vi "sub_ofdm_simple_delayed_mult_CFO_sync_single.vi"(8 "CP length":i32=64, 9 "FFT size":i32=256, 11 "time samples":cdb[](array[numeric])) -> (3 "sync ofdm symbol":cdb[](array[numeric]))   [LabVIEW 2014]
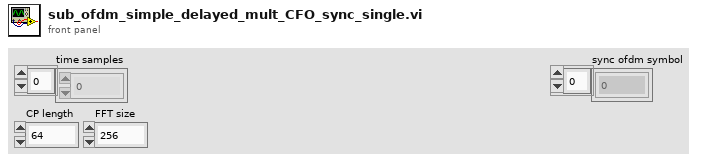
[diagram p1: front panel]
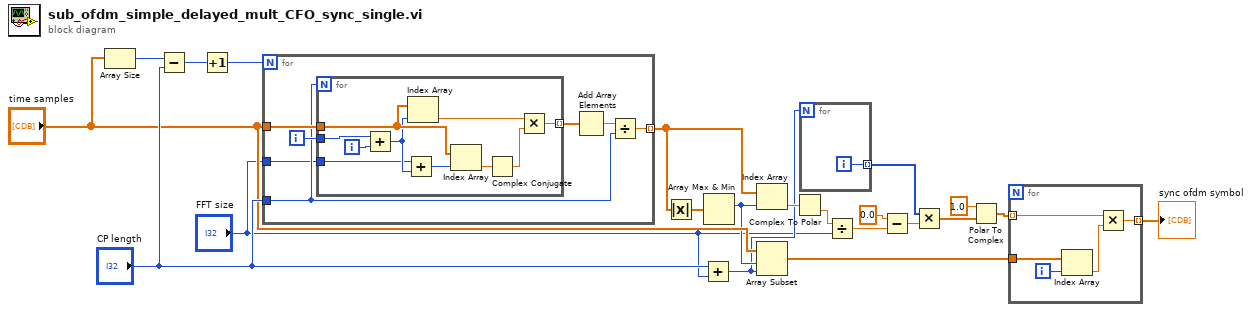
[diagram p0: block diagram]
diagram:
  n1 = Array Size(array="time samples") -> (size(s)=w17:i32)
  n2 = Subtract(x=w17, y="CP length") -> (x-y=w16:i32)
  n3 = Increment(x=w16) -> (x+1=w15:i32)
  n4 = for {
    N: w15 -> [_]
    tunnel: "CP length" -> [w26]
    tunnel: "time samples" -> [w28]
    tunnel: [w23] -> w20 mode=indexing
    tunnel: "FFT size" -> [w22]
    i -> [w27]
    n5 = for {
      N: w26 -> [_]
      tunnel: w28 -> [w34]
      tunnel: w27 -> [w38]
      tunnel: [w30] -> w24 mode=indexing
      tunnel: w22 -> [w29]
      i -> [w37]
      n6 = Add(x=w38, y=w37) -> (x+y=w33:i32)
      n7 = Add(x=w29, y=w33) -> (x+y=w36:i32)
      n8 = Index Array(array=w34, index=w33) -> (element=w32:cdb)
      n9 = Index Array(array=w34, index=w36) -> (element=w35:cdb)
      n10 = Complex Conjugate(1:w35) -> (0:w31:cdb)
      n11 = Multiply(x=w32, y=w31) -> (x*y=w30:cdb)
    }
    n12 = Add Array Elements(numeric array=w24) -> (sum=w25:cdb)
    n13 = Divide(x=w25, y=w26) -> (x/y=w23:cdb)
  }
  n14 = Absolute Value(x=w20) -> (abs(x)=w21:dbl[])
  n15 = Add(x="CP length", y="FFT size") -> (x+y=w11:i32)
  n16 = Array Max & Min(array=w21) -> (max index (indices)=w12:i32)  [unwired: 3 out]
  n17 = Index Array(array=w20, index=w12) -> (element=w18:cdb)
  n18 = Array Subset(array="time samples", index=w12, length=w11) -> (w4:cdb[])
  n19 = Complex To Polar(r * e^(i*theta)=w18) -> (theta=w19:dbl)  [unwired: 1 out]
  n20 = for {
    N: w11 -> [_]
    tunnel: [w39] -> w9 mode=indexing
    i -> [w39]
  }
  n21 = Divide(x=w19, y="FFT size") -> (x/y=w5:dbl)
  n22 = Subtract(x=0.0, y=w5) -> (x-y=w8:dbl)
  n23 = Multiply(x=w9, y=w8) -> (x*y=w7:dbl[])
  n24 = Polar To Complex(1:w7, 2:1.0) -> (0:w6:cdb[])
  n25 = for {
    tunnel: w6 -> [w41] mode=indexing
    tunnel: w4 -> [w44]
    tunnel: [w40] -> w3 mode=indexing
    i -> [w43]
    n26 = Index Array(array=w44, index=w43) -> (element=w42:cdb)
    n27 = Multiply(x=w41, y=w42) -> (x*y=w40:cdb)
  }
  "sync ofdm symbol" <- w3
